vi "Plugin Options Panel Start.vi"(6 "Index in":i32, 8 "error in (no error)":errorcluster, 10 "Container":refnum<vi>, 11 "Plugins in":refnum<class "Plugin.lvclass">[](array[class])) -> (0 "error out":errorcluster, 1 "Config VI Refnum out":refnum<vi>, 3 "Plugins out":refnum<class "Plugin.lvclass">[](array[class]))   [LabVIEW 2015, in "Application.lvclass"]
uses:
  Application.lvclass
  Plugin.lvclass
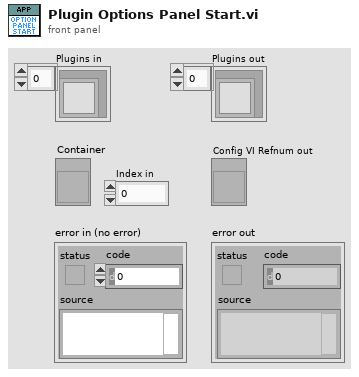
[diagram p1: front panel]
types:
  T1 = enum32{"Invalid", "Standard", "Closed", "Hidden", "Minimized", "Maximized"}
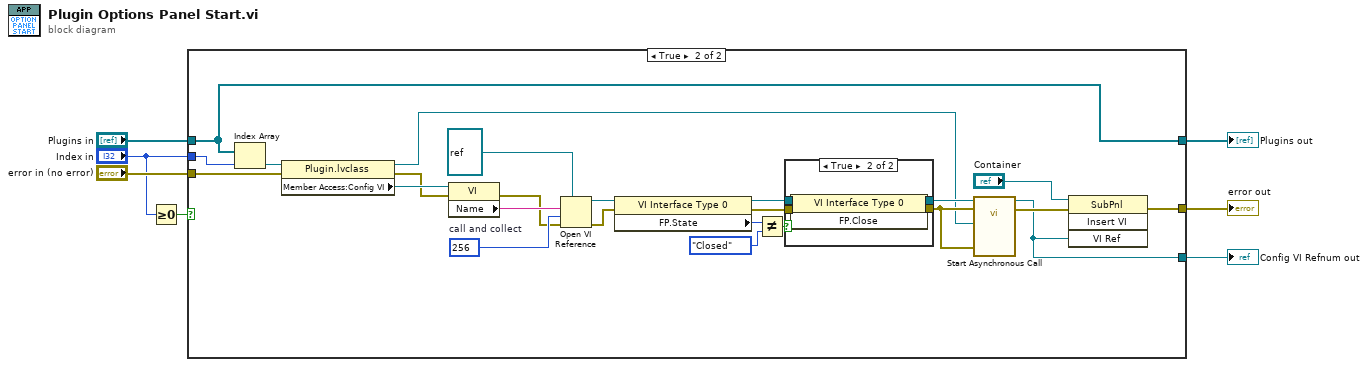
[diagram p0: block diagram]
diagram:
  n1 = Greater Or Equal To 0?(x="Index in") -> (x >= 0?=w2:bool)
  n2 = case shown="True" w2 {
    tunnel: [_ w19] -> w7
    tunnel: "error in (no error)" -> [w9 w16]
    tunnel: [w9 w15] -> w5
    tunnel: "Plugins in" -> [w8 w10]
    tunnel: "Index in" -> [_ w11]
    tunnel: [w8 w10] -> w1
    frame False {
    }
    frame True {
      w31 = 256  # call and collect
      n3 = Index Array(array=w10, index=w11) -> (element=w12:refnum<class "Plugin.lvclass">)
      n4 = property class="Plugin.lvclass"(reference=w12, error in=w16) -> (reference out=w13:refnum<class "Plugin.lvclass">, error out=w17:errorcluster, "Member Access:Config VI"=w18:refnum<vi>)
      n5 = property class="VI"(reference=w18, error in=w17) -> (error out=w30:errorcluster, "Name"=w32:string)  [unwired: 1 out]
      n6 = Open VI Reference(type specifier VI Refnum (for type only)=refnum<vi> refnum, vi path=w32, options=w31, error in (no error)=w30) -> (vi reference=w24:refnum<vi>, error out=w23:errorcluster)  [unwired: 2 in]
      n7 = property class="VI Interface Type 0"(reference=w24, error in=w23) -> (reference out=w28:refnum<vi>, error out=w29:errorcluster, "FP.State"=w25:T1)
      n8 = Not Equal?(x=w25, y=T1."Closed" ("Front Panel Window:State")) -> (x != y?=w27:bool)
      n9 = case shown="True" w27 {
        tunnel: w28 -> [w35 w39]
        tunnel: w29 -> [w34 w38]
        tunnel: [w35 w37] -> w22
        tunnel: [w34 w36] -> w21
        frame False {
        }
        frame True {
          n10 = invoke class="VI Interface Type 0" method="FP.Close"(reference=w39, error in=w38) -> (reference out=w37:refnum<vi>, error out=w36:errorcluster)  [unwired: 1 in, 1 out]
        }
      }
      n11 = call-by-ref "Start Asynchronous Call"(reference=w22, error in=w21, 8:"error in (no error)"=w21, "Plugin in"=w13) -> (reference out=w19:refnum<vi>, error out=w20:errorcluster)  [unwired: 8 in, 2 out]
      n12 = invoke class="SubPnl" method="Insert VI"(reference="Container", error in=w20, "VI Ref"=w19) -> (error out=w15:errorcluster)  [unwired: 1 in, 3 out]
    }
  }
  "error out" <- w5
  "Config VI Refnum out" <- w7
  "Plugins out" <- w1
